vi "RANGE General Factors.vi"(8 "Error In":errorcluster, 11 "Gas Type String":string) -> (0 "Error Out":errorcluster, 2 "Flow Rate Factor":dbl)   [LabVIEW 2018]
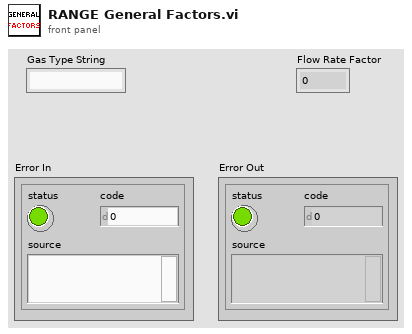
[diagram p1: front panel]
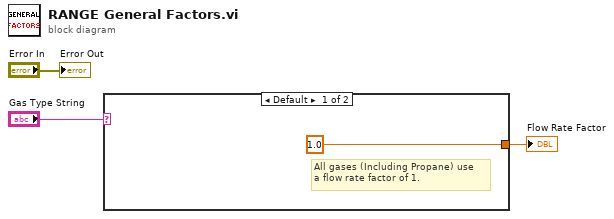
[diagram p0: block diagram]
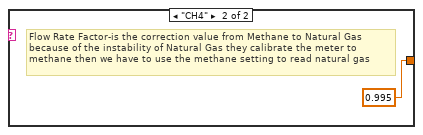
[diagram p2: hidden frame]
diagram:
  n1 = case shown="Default" "Gas Type String" {
    tunnel: [1.0 0.995] -> w3
    frame Default {
      # "All gases (Including Propane) use\na flow rate factor of 1."
    }
    frame "CH4" {
      # "Flow Rate Factor-is the correction value from Methane to Natural Gas\nbecause of the instability of Natural Gas they calibrate the meter to\nmethane then we have to use the methane setting to read natural gas"
    }
  }
  "Flow Rate Factor" <- w3
  "Error Out" <- "Error In"
